vi "Servo State FGV.vi"(2 "error in (no error)":errorcluster, 3 "Init/Read/Write State":T2=enum."Write", 4 "Servo State":T1) -> (0 "error out":errorcluster, 1 "Output":dbl)   [LabVIEW 2018]
uses:
  Labview Training Phase 2/Enum Controls/States for Action Engine.ctl
  Servo States FGV Enum.ctl
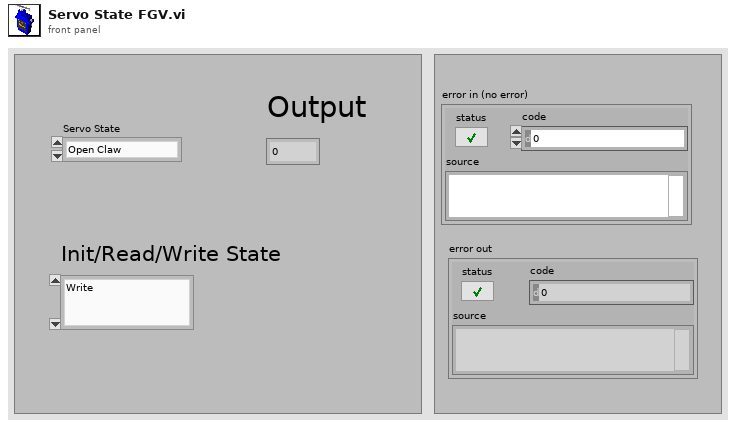
[diagram p1: front panel]
types:
  T1 = typedef "Servo States FGV Enum.ctl" = enum16{"Open Claw", "Close claw"}
  T2 = typedef "States for Action Engine.ctl" = enum16{"Initialize", "Write", "Read"}
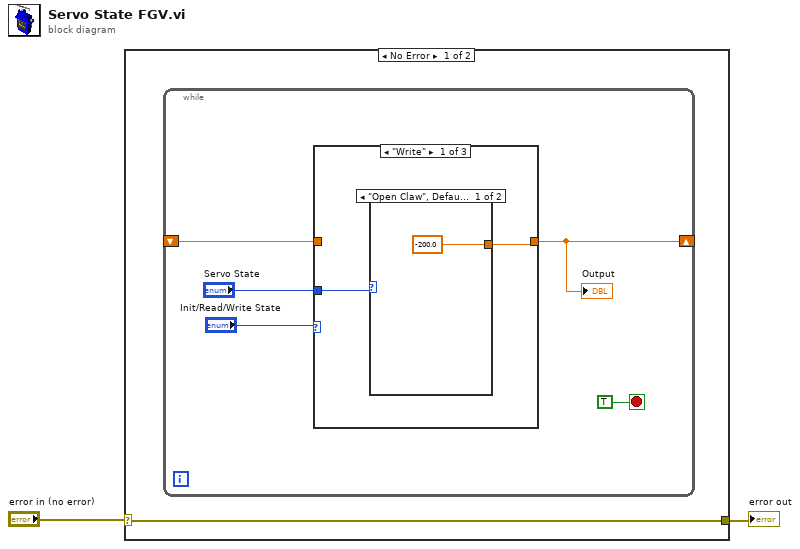
[diagram p0: block diagram]
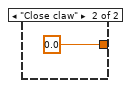
[diagram p2: hidden frame]
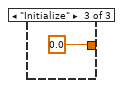
[diagram p4: hidden frame]
diagram:
  n1 = case shown="No Error" "error in (no error)" {
    selector: "error in (no error)" -> [w3 w15]
    tunnel: [w3 w15] -> w1
    frame No Error {
      n2 = while {
        shift-right: [w5] -> _
        shift-left: _ -> [w6]
        stop <- TRUE stop-if-true
        n3 = case shown="\"Write\"" "Init/Read/Write State" {
          tunnel: [w9 w13 0.0] -> w5
          tunnel: w6 -> [_ w13 _]
          tunnel: "Servo State" -> [w10 _ _]
          frame "Write" {
            n4 = case shown="\"Open Claw\", Default" w10 {
              tunnel: [-200.0 0.0] -> w9
              frame "Open Claw", Default {
              }
              frame "Close claw" {
              }
            }
          }
          frame "Read", Default {
            # "In this state, the output \nvalue is read from \nthe shift register"
          }
          frame "Initialize" {
          }
        }
        "Output" <- w5
      }
    }
    frame Error {
    }
  }
  "error out" <- w1
